vi "LJM_UINT16ToByteArray.vi"(1 "U16":u16) -> (0 "Byte Array":u8[](array[numeric]))   [LabVIEW 2024]
panel:
  # "Converts a U16 to a 2-element big-endian byte array."
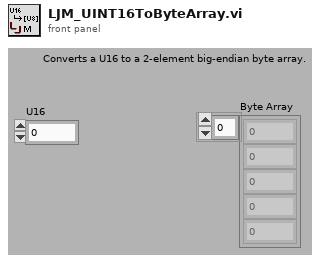
[diagram p1: front panel]
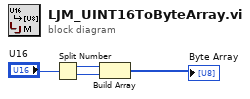
[diagram p0: block diagram]
diagram:
  n1 = Split Number(x="U16") -> (hi(x)=w3:u8, lo(x)=w2:u8)
  n2 = Build Array(w3, w2) -> (→"Byte Array":u8[])
